vi "5668 Configure Power Level.vi"(8 "error in (no error)":errorcluster, 10 "reference level (dBm)":dbl caption="Reference Level (dBm)" format="%.2f", 11 "Instrument Handles in":T1={"Resource Name RFSA"="RFSA", "Resource Name RFSG LO Generation"="RFSG"}) -> (0 "error out":errorcluster, 3 "Instrument Handles out":T1={"Resource Name RFSA"="RFSA", "Resource Name RFSG LO Generation"="RFSG"})   [LabVIEW 2017]
uses:
  Instrument Handles.ctl
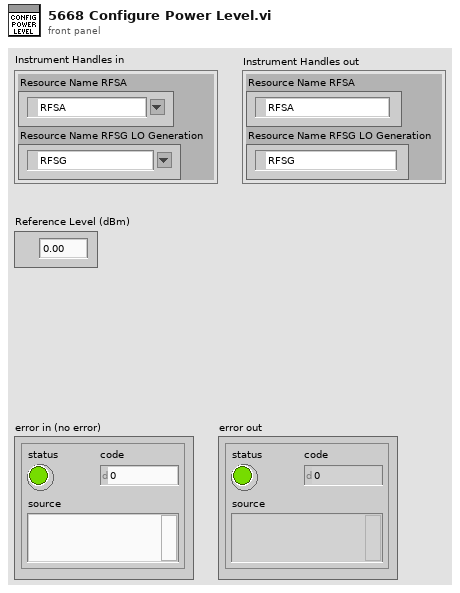
[diagram p1: front panel]
types:
  T1 = typedef "Instrument Handles.ctl" = cluster{"Resource Name RFSA":refnum<k15>, "Resource Name RFSG LO Generation":refnum<k15>}
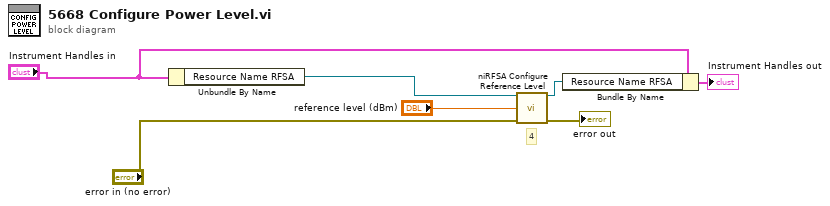
[diagram p0: block diagram]
diagram:
  # "4"
  n1 = Unbundle By Name("Instrument Handles in") -> ("Resource Name RFSA"=w5:refnum<k15>)
  n2 = call <instrlib>:"niRFSA Configure Reference Level.vi"("instrument handle"=w5, "reference level (dBm)"="reference level (dBm)", "error in"="error in (no error)") -> ("instrument handle out"=w4:refnum<k15>, "error out"=→"error out":errorcluster)  [unwired: 11 in]
  n3 = Bundle By Name(cluster="Instrument Handles in", "Resource Name RFSA"=w4) -> (→"Instrument Handles out":T1)
